vi "Read Resolved File Path.vi"(8 "error in (no error)":errorcluster, 11 "File Handler in":refnum<class "File Handler.lvclass">) -> (0 "error out":errorcluster, 2 "Resolved File Path":path, 3 "File Handler out":refnum<class "File Handler.lvclass">)   [LabVIEW 2018, in "GLog.lvlib" / "File Handler.lvclass"]
uses:
  <vilib>/NQE/GLog/src/api/configuration/handlers/file_handler/File Handler.lvclass
  <vilib>/NQE/GLog/src/api/configuration/handlers/file_handler/File Handler.lvclass/File Handler.ctl
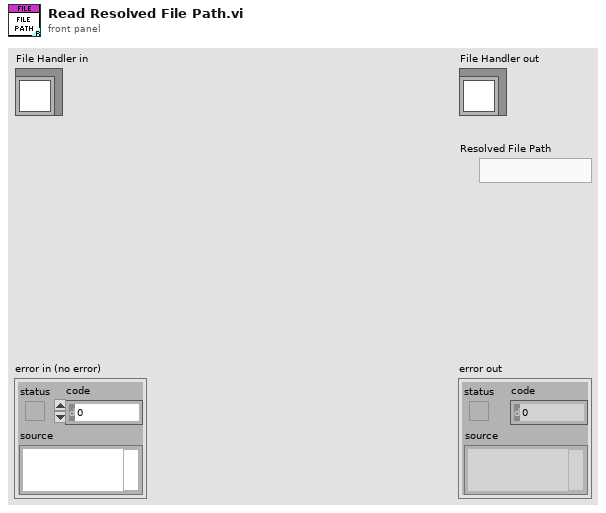
[diagram p1: front panel]
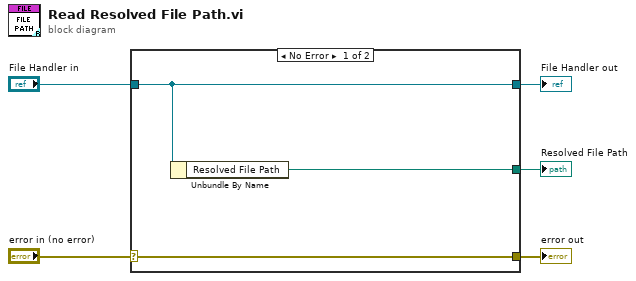
[diagram p0: block diagram]
diagram:
  n1 = case shown="No Error" "error in (no error)" {
    selector: "error in (no error)" -> [w8 w9]
    tunnel: [w8 w9] -> w4
    tunnel: [w7 w10] -> w2
    tunnel: "File Handler in" -> [w7 w10]
    tunnel: [w6 _] -> w1
    frame No Error {
      n2 = Unbundle By Name(w7) -> ("Resolved File Path"=w6:path)
    }
    frame Error {
    }
  }
  "error out" <- w4
  "File Handler out" <- w2
  "Resolved File Path" <- w1
